vi "SB_piston_stuck.vi"(8 "error in (no error)":errorcluster) -> (0 "error out":errorcluster)   [LabVIEW 2013]
uses:
  My Computer/Controls/Advanced Swimbladder Indicators.ctl
  My Computer/Controls/Sensors State.ctl
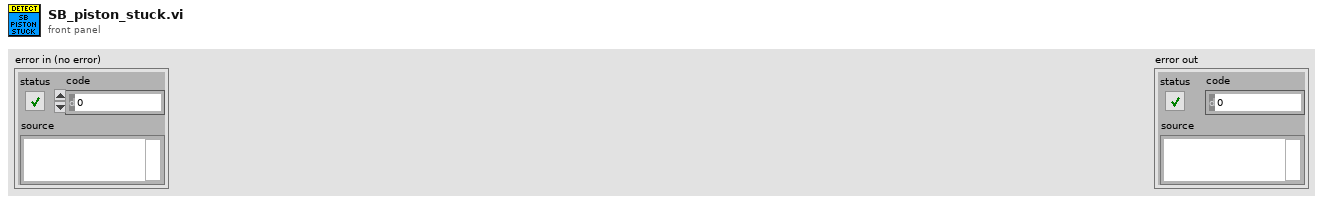
[diagram p1: front panel]
types:
  T1 = typedef "Advanced Swimbladder Indicators.ctl" = cluster{"P_ref [Pa]":dbl, "X_Actual [m]":dbl, "Motor Current[A]":dbl}
  T2 = typedef "Sensors State.ctl" = cluster{"Leakage-Sensor_enabled":bool, "IMU_enabled":bool, "Swimbladder Fill-State-Sensor_enabled":bool, "Flow-Sensor_enabled":bool, "Depth-Sensor_enabled":bool, "Current-Sensor_enabled":bool, "Calibrate Depth":bool, "SB_Piston_Stuck_Detect_enabled":bool, "Check_too_Deep_enabled":bool}
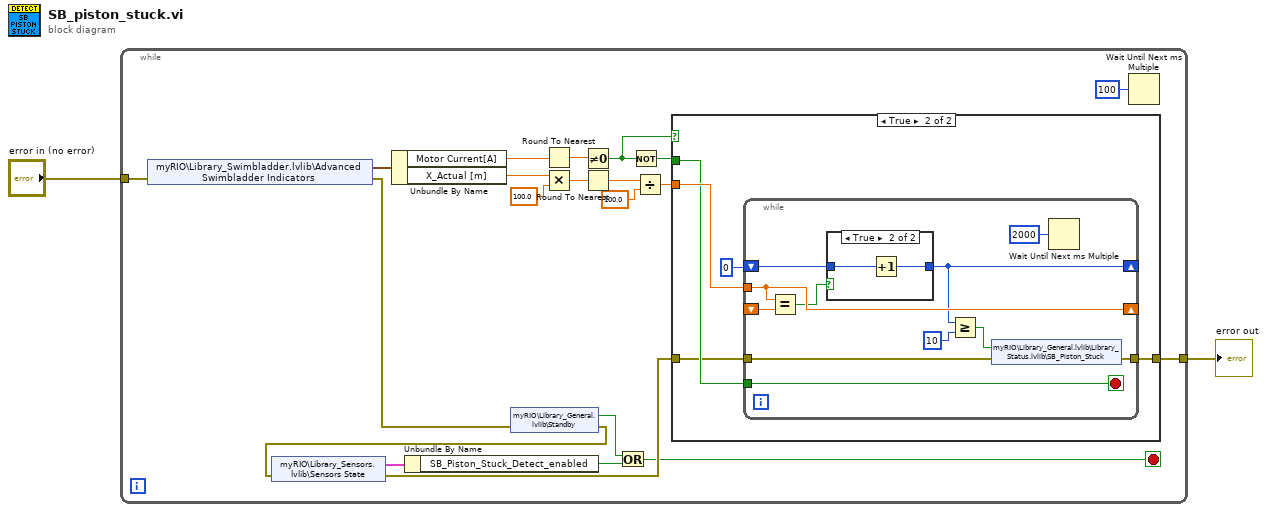
[diagram p0: block diagram]
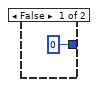
[diagram p3: hidden frame]
diagram:
  n1 = while {
    tunnel: "error in (no error)" -> [w23]
    tunnel: [w17] -> w1
    stop <- w9 stop-if-true
    n2 = shared-variable "myRIO\\Library_Swimbladder.lvlib\\Advanced Swimbladder Indicators"(error in=w23) -> (w22:T1, error out=w15:errorcluster)
    n3 = Unbundle By Name(w22) -> ("Motor Current[A]"=w19:dbl, "X_Actual [m]"=w8:dbl)
    n4 = shared-variable "myRIO\\Library_General.lvlib\\Standby"(error in=w15) -> (w11:bool, error out=w13:errorcluster)
    n5 = shared-variable "myRIO\\Library_Sensors.lvlib\\Sensors State"(error in=w13) -> (w14:T2, error out=w12:errorcluster)
    n6 = Unbundle By Name(w14) -> ("SB_Piston_Stuck_Detect_enabled"=w10:bool)
    n7 = Round To Nearest(number=w19) -> (nearest integer value=w18:dbl)
    n8 = Multiply(x=w8, y=100.0) -> (x*y=w6:dbl)
    n9 = Not Equal To 0?(x=w18) -> (x != 0?=w21:bool)
    n10 = Round To Nearest(number=w6) -> (nearest integer value=w5:dbl)
    n11 = Or(x=w11, y=w10) -> (x .or. y?=w9:bool)
    n12 = Not(x=w21) -> (.not. x?=w20:bool)
    n13 = Divide(x=w5, y=100.0) -> (x/y=w3:dbl)
    n14 = case shown="True" w21 {
      tunnel: w3 -> [_ w29]
      tunnel: w20 -> [_ w27]
      tunnel: w12 -> [w24 w26]
      tunnel: [w24 w25] -> w17
      frame False {
      }
      frame True {
        n15 = while {
          tunnel: w29 -> [w40]
          shift-right: [w40] -> _
          shift-left: _ -> [w39]
          shift-right: [w35] -> _
          shift-left: i8 0 ("x") -> [w37]
          tunnel: w27 -> [w33]
          tunnel: w26 -> [w31]
          tunnel: [w30] -> w25
          stop <- w33 stop-if-true
          n16 = Equal?(x=w40, y=w39) -> (x = y?=w38:bool)
          n17 = case shown="True" w38 {
            tunnel: w37 -> [_ w43]
            tunnel: [i8 0 w42] -> w35
            frame False {
            }
            frame True {
              n18 = Increment(x=w43) -> (x+1=w42:i8)
            }
          }
          n19 = Greater Or Equal?(x=w35, y=i8 10) -> (x >= y?=w32:bool)
          n20 = shared-variable "myRIO\\Library_General.lvlib\\Library_Status.lvlib\\SB_Piston_Stuck"(w32, error in=w31) -> (error out=w30:errorcluster)
          n21 = Wait Until Next ms Multiple(millisecond multiple=u32 2000) -> ()  [unwired: 1 out]
        }
      }
    }
    n22 = Wait Until Next ms Multiple(millisecond multiple=u32 100) -> ()  [unwired: 1 out]
  }
  "error out" <- w1
